vi "Car Wash.vi"() -> ()   [LabVIEW 2015]
uses:
  controls/Car Wash Indicators.ctl
  controls/Wash Options.ctl
  controls/UI Data.ctl
  support/Message Queue/Enqueue Message (Single).vi
  <vilib>/Utility/error.llb/Error Cluster From Error Code.vi
  <vilib>/ErrorRing/Error Ring.xnode
  support/Message Queue/Message Queue.lvlib
  support/User Event - Stop/User Event - Stop.lvlib
panel:
  in  "Start":bool
  out "Elapsed Time":dbl format="%0.2f"
  in  "stop":bool
  out "Wash Entry":bool
  in  "Wash Options":T1
  in  "Car Position Slider":u8(slide) max=3 scale=0.0..4.0
  out "Car Wash Indicators":T2
  # "Entry Console"
  # "Car Wash Display"
  # "Car Position Simulation"
  # "Pre-Soak\nH-P Wash\nL-P Wax\nSpot Free Rinse"
  # "Underbody Wash\nBug Remover"
  # "Tire Shine\nAir Dry"
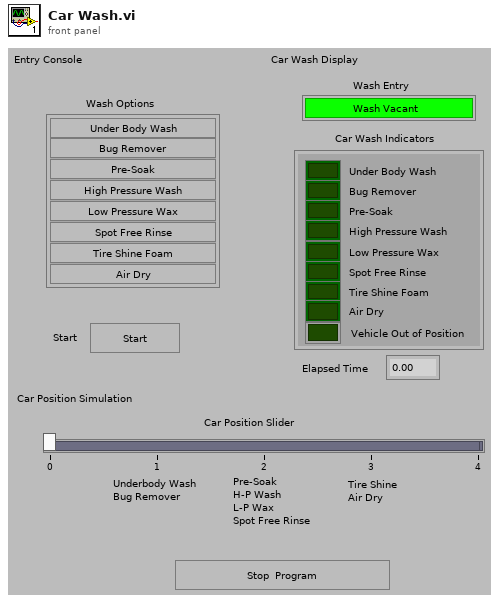
[diagram p1: front panel]
types:
  T1 = typedef "Wash Options.ctl" = cluster{"Underbody Wash":bool, "Bug Remover":bool, "Pre-Soak":bool, "High Pressure Wash":bool, "Low Pressure Wax":bool, "Spot Free Rinse":bool, "Tire Shine Foam":bool, "Air Dry":bool}
  T2 = typedef "Car Wash Indicators.ctl" = cluster{"Under Body Wash":bool, "Bug Remover":bool, "Pre-Soak":bool, "High Pressure Wash":bool, "Low Pressure Wax":bool, "Spot Free Rinse":bool, "Tire Shine Foam":bool, "Air Dry":bool, "Vehicle Out of Position":bool}
  T3 = typedef "UI Data.ctl" = cluster{"Underbody Wash Ref":refnum<vi>, "Bug Remover Ref":refnum<vi>, "Pre-Soak Ref":refnum<vi>, "High Pressure Wash Ref":refnum<vi>, "Low Pressure Wax Ref":refnum<vi>, "Spot Free Rinse Ref":refnum<vi>, "Tire Shine Foam Ref":refnum<vi>, "Air Dry Ref":refnum<vi>}
  T4 = typedef "Message Queue.lvlib/All Message Queues.ctl" = cluster{"UI":refnum<queue>}
  T5 = enum8{"Enabled", "Disabled", "Disabled and Grayed Out"}
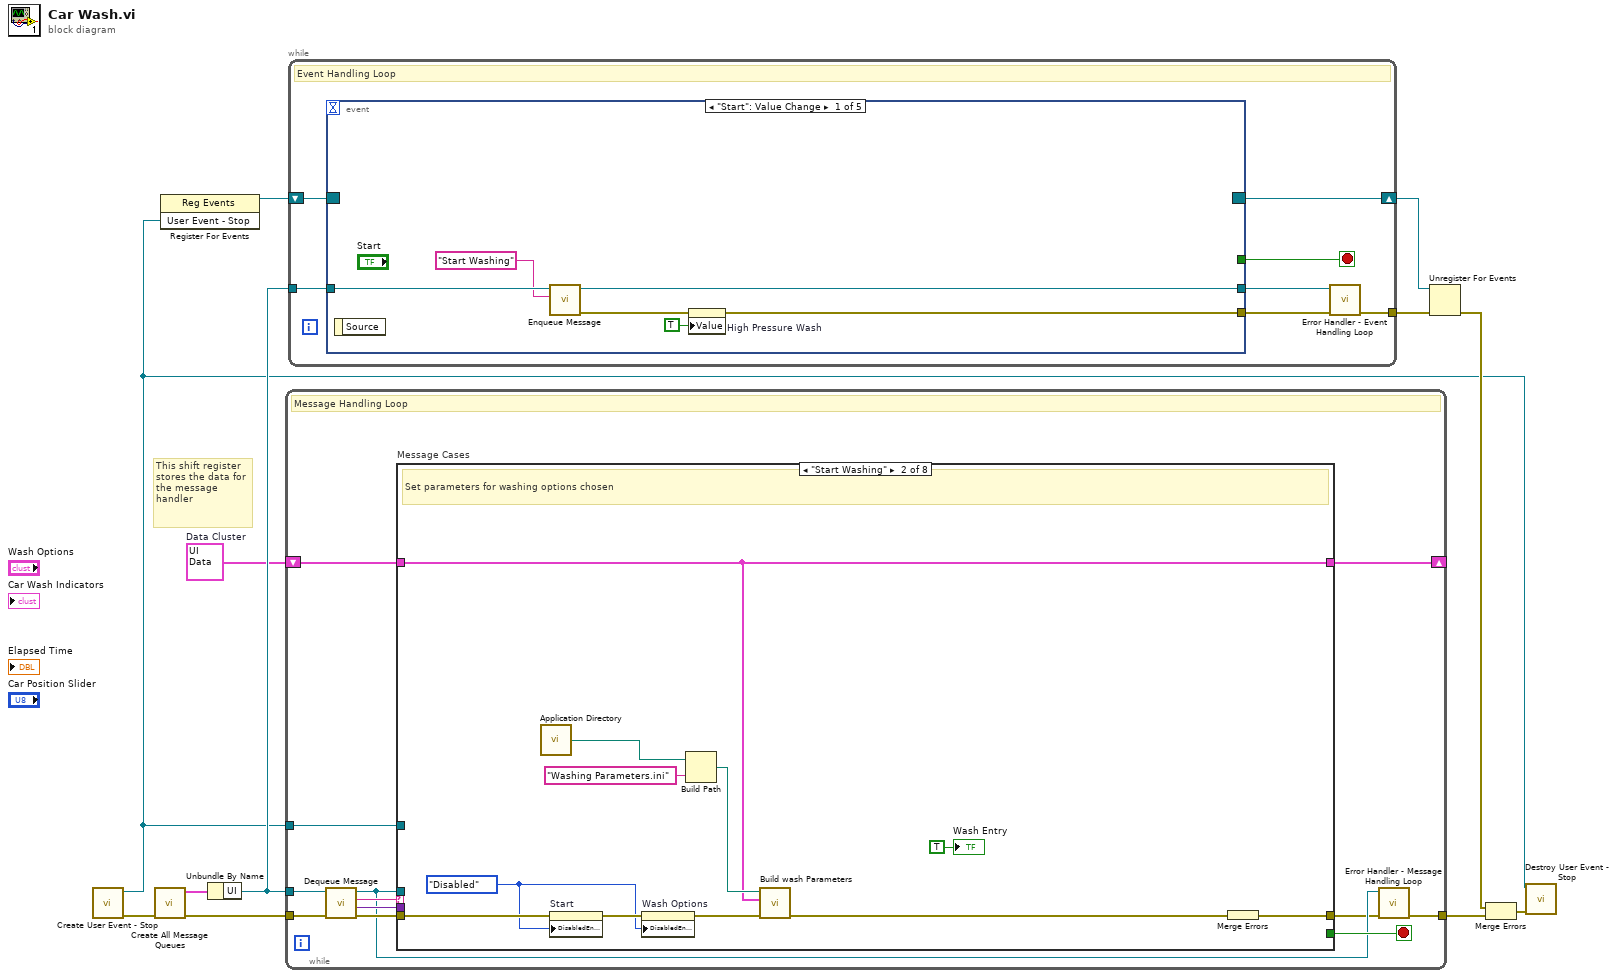
[diagram p0: block diagram]
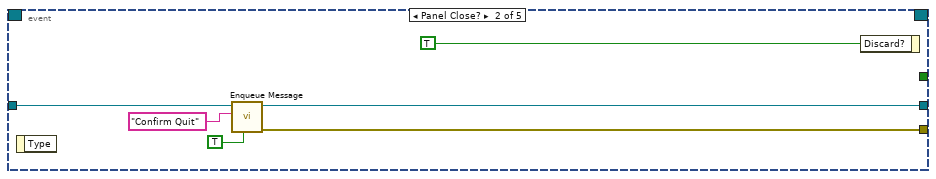
[diagram p2: hidden frame]
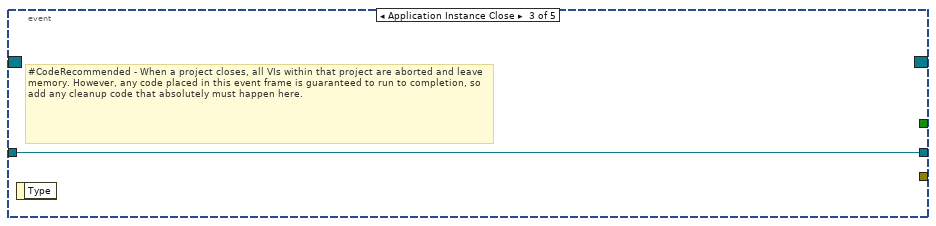
[diagram p3: hidden frame]
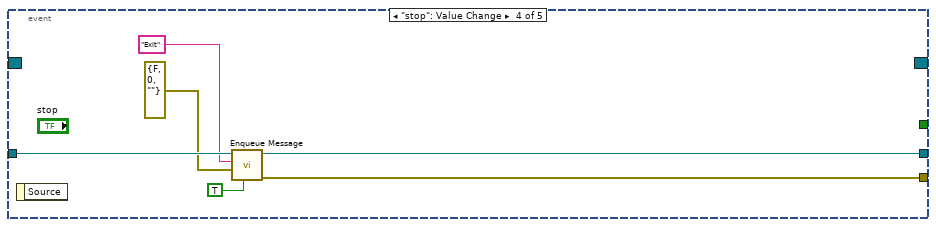
[diagram p4: hidden frame]
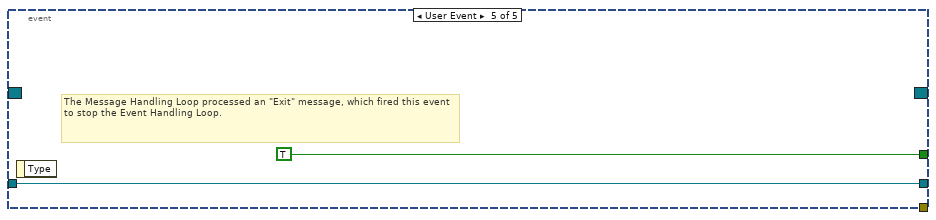
[diagram p5: hidden frame]
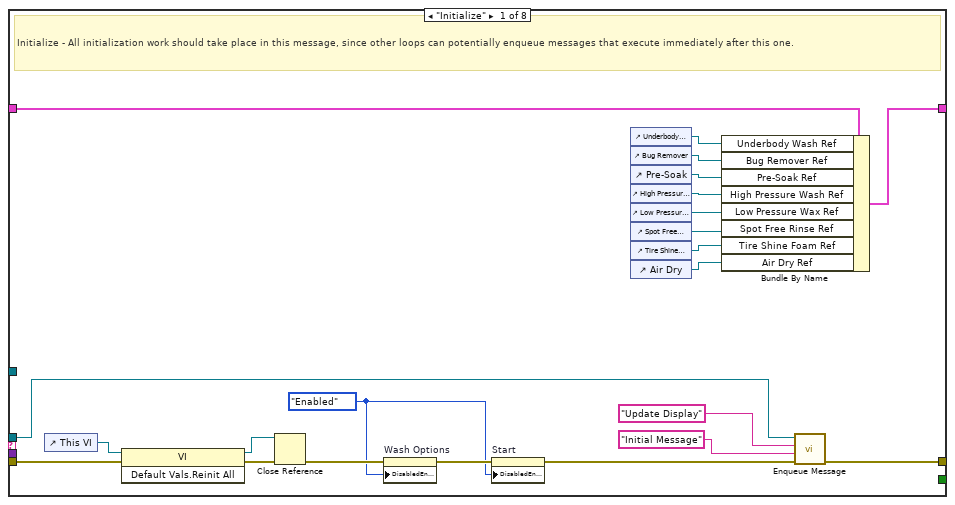
[diagram p6: hidden frame]
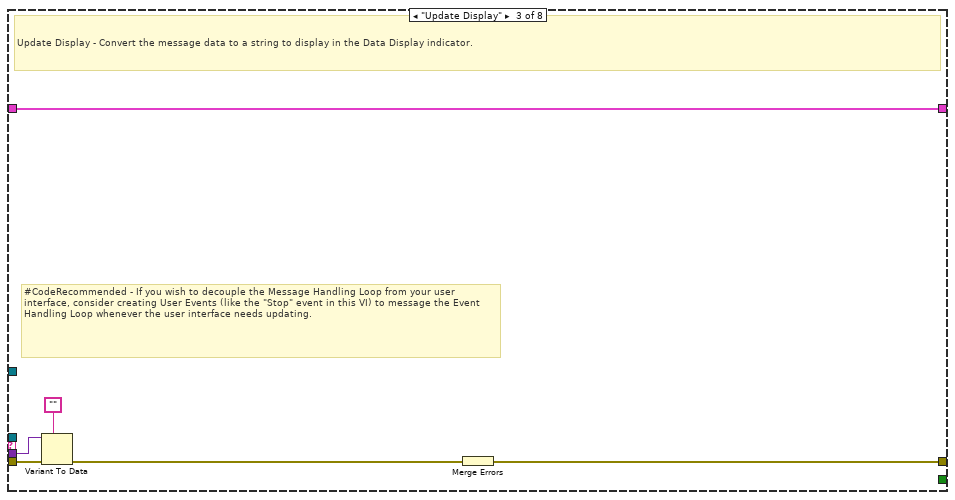
[diagram p7: hidden frame]
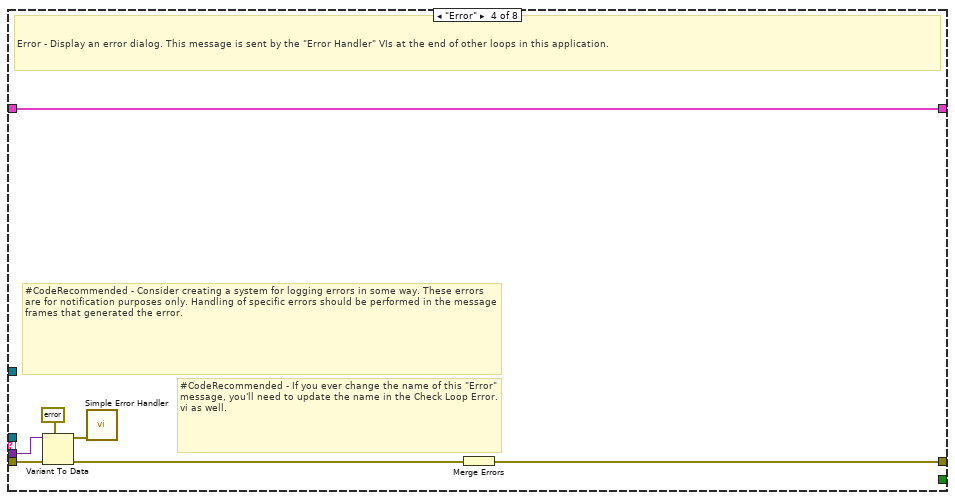
[diagram p8: hidden frame]
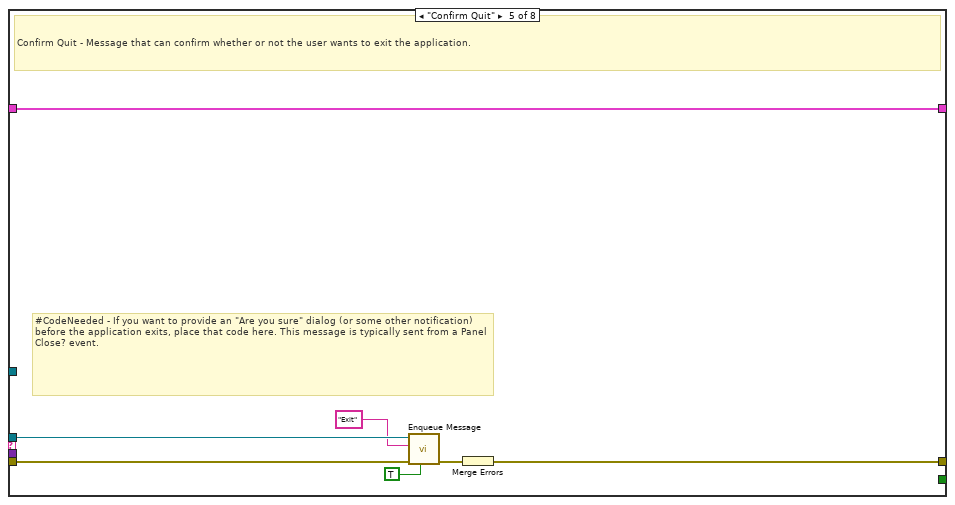
[diagram p9: hidden frame]
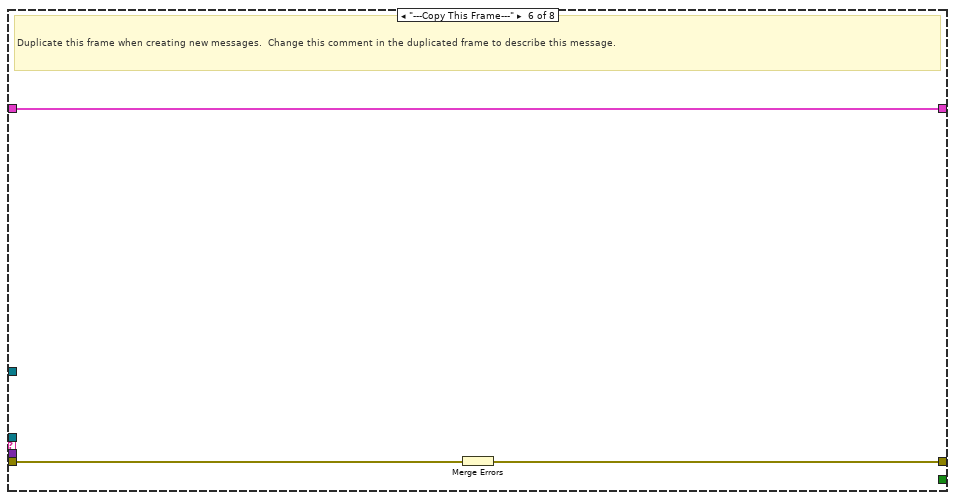
[diagram p10: hidden frame]
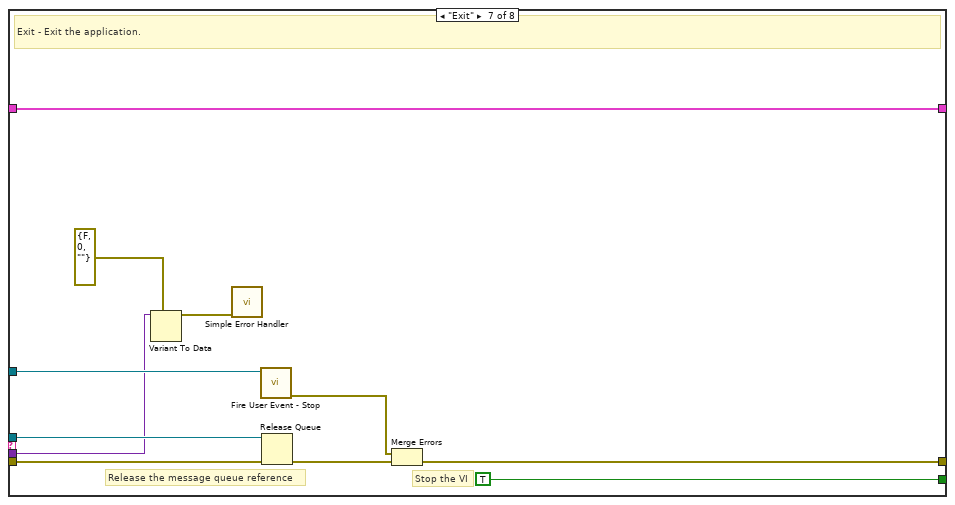
[diagram p11: hidden frame]
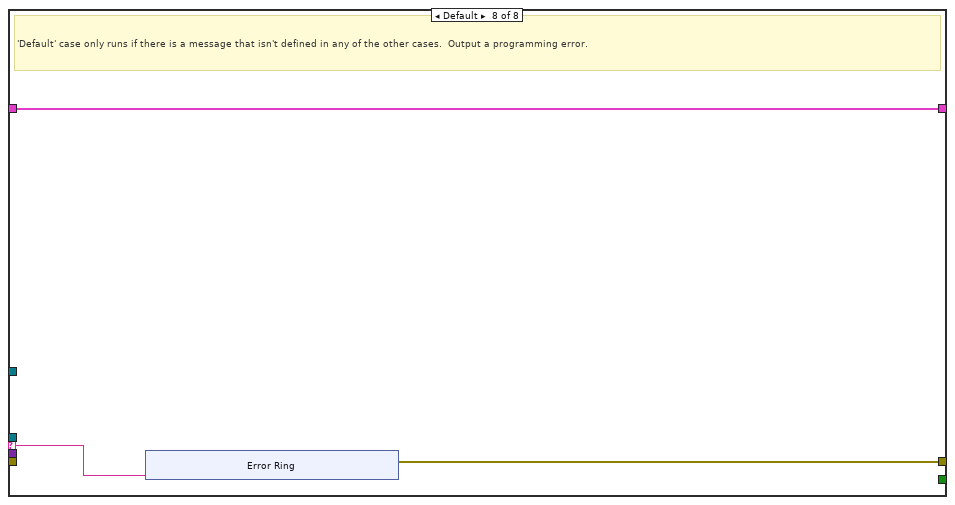
[diagram p12: hidden frame]
diagram:
  w4 = T3 {"Underbody Wash Ref"=refnum, "Bug Remover Ref"=refnum, "Pre-Soak Ref"=refnum, "High Pressure Wash Ref"=refnum, "Low Pressure Wax Ref"=refnum, "Spot Free Rinse Ref"=refnum, "Tire Shine Foam Ref"=refnum, "Air Dry Ref"=refnum}  # Data Cluster
  # "This shift register stores the data for the message handler"
  n1 = call "Create User Event - Stop.vi"() -> ("error out"=w8:errorcluster, "User Event - Stop"=w1:refnum<user-event>)  [unwired: 10 in]
  n2 = call "Create All Message Queues.vi"("error in (no error)"=w8) -> ("error out"=w12:errorcluster, "Message Queues out"=w11:T4)  [unwired: 9 in]
  n3 = register-events(w1) -> (reference out=w2:refnum<event-registration>)  [unwired: 2 in, 1 out]
  n4 = Unbundle By Name(w11) -> ("UI"=w9:refnum<queue>)
  n5 = while {
    tunnel: w9 -> [w16]
    shift-right: [w23] -> _
    shift-left: w4 -> [w24]
    tunnel: w1 -> [w21]
    tunnel: w12 -> [w20]
    tunnel: [w14] -> w10
    stop <- w22 stop-if-true
    # "Message Handling Loop"
    n6 = call "Dequeue Message.vi"("error in (no error)"=w20, "Message Queue"=w16) -> ("error out"=w19:errorcluster, "Message Data"=w17:variant, "Message"=w18:string, "dup Message Queue"=w15:refnum<queue>)  [unwired: 6 in]
    n7 = case "Message Cases" shown="\"Start Washing\"" w18 {
      selector: w18 -> [_ _ _ _ _ _ _ w92]
      tunnel: w15 -> [w44 _ _ _ w73 _ w91 _]
      tunnel: w19 -> [w31 w49 w61 w70 w77 w80 w84 _]
      tunnel: [w46 w57 w62 w64 w75 w78 w87 w93] -> w13
      tunnel: w24 -> [w34 w53 w63 w69 w76 w79 w90 w94]
      tunnel: [w33 w53 w63 w69 w76 w79 w90 w94] -> w23
      tunnel: [_ _ _ _ _ _ TRUE _] -> w22
      tunnel: w17 -> [_ _ w60 w68 _ _ w82 _]
      tunnel: w21 -> [_ _ _ _ _ _ w86 _]
      frame "Initialize" {
        w26 = T5."Enabled" ("Disabled")
        # "Initialize - All initialization work should take place in this message, since other loops can potentially enqueue messages that execute immediately after this one."
        n8 = control-ref of="This VI"() -> (w32:refnum<vi>)
        n9 = invoke class="VI" method="Default Vals.Reinit All"(reference=w32, error in=w31) -> (reference out=w30:refnum<vi>, error out=w29:errorcluster)  [unwired: 1 in, 1 out]
        n10 = Close Reference(reference=w30, error in (no error)=w29) -> (error out=w28:errorcluster)
        n11 = property on="Wash Options" class="Clust (strict)"(error in=w28, "DisabledEnum"=w26) -> (error out=w27:errorcluster)  [unwired: 1 in, 1 out]
        n12 = property on="Start" class="Bool"(error in=w27, "DisabledEnum"=w26) -> (error out=w25:errorcluster)  [unwired: 1 in, 1 out]
        n13 = control-ref of="Underbody Wash"() -> (w42:refnum<vi>)
        n14 = control-ref of="Bug Remover"() -> (w41:refnum<vi>)
        n15 = control-ref of="Pre-Soak"() -> (w40:refnum<vi>)
        n16 = control-ref of="High Pressure Wash"() -> (w39:refnum<vi>)
        n17 = control-ref of="Low Pressure Wax"() -> (w38:refnum<vi>)
        n18 = control-ref of="Spot Free Rinse"() -> (w37:refnum<vi>)
        n19 = control-ref of="Tire Shine Foam"() -> (w36:refnum<vi>)
        n20 = control-ref of="Air Dry"() -> (w35:refnum<vi>)
        n21 = Bundle By Name(cluster=w34, "Underbody Wash Ref"=w42, "Bug Remover Ref"=w41, "Pre-Soak Ref"=w40, "High Pressure Wash Ref"=w39, "Low Pressure Wax Ref"=w38, "Spot Free Rinse Ref"=w37, "Tire Shine Foam Ref"=w36, "Air Dry Ref"=w35) -> (w33:T3)
        n22 = call-poly "Enqueue Message.vi"("error in (no error)"=w25, "Message Data"="Initial Message" ("Initial Message"), "Message"="Update Display", "Message Queue"=w44) -> ("error out"=w46:errorcluster)  [unwired: 6 in, 1 out]
      }
      frame "Start Washing" {
        w48 = T5."Disabled" ("Disabled")
        # "Set parameters for washing options chosen"
        n23 = call <vilib>:"Application Directory.vi"() -> ("Application Directory"=w56:path)
        n24 = property on="Start" class="Bool"(error in=w49, "DisabledEnum"=w48) -> (error out=w50:errorcluster)  [unwired: 1 in, 1 out]
        n25 = property on="Wash Options" class="Clust (strict)"(error in=w50, "DisabledEnum"=w48) -> (error out=w51:errorcluster)  [unwired: 1 in, 1 out]
        n26 = Build Path(base path=w56, name or relative path="Washing Parameters.ini") -> (appended path=w54:path)
        n27 = call "Build wash Parameters.vi"("error in (no error)"=w51, "Data Controls"=w53, "configuration file path"=w54) -> ("error out"=w52:errorcluster)  [unwired: 7 in, 1 out]
        n28 = Merge Errors(w52) -> (w57:errorcluster)
        "Wash Entry" <- TRUE ("Wash Entry")
      }
      frame "Update Display" {
        # "#CodeRecommended - If you wish to decouple the Message Handling Loop from your user interface, consider creating User Events (like the \"Stop\" event in this VI) to message the Event Handling Loop whenever the user interface needs updating."
        # "Update Display - Convert the message data to a string to display in the Data Display indicator."
        n29 = Variant To Data(error in=w61, type="", Variant=w60) -> (error out=w58:errorcluster)  [unwired: 1 out]
        n30 = Merge Errors(w58) -> (w62:errorcluster)
      }
      frame "Error" {
        # "#CodeRecommended - If you ever change the name of this \"Error\" message, you'll need to update the name in the Check Loop Error.vi as well."
        # "#CodeRecommended - Consider creating a system for logging errors in some way. These errors are for notification purposes only. Handling of specific errors should be performed in the message frames that generated the error."
        # "Error - Display an error dialog. This message is sent by the \"Error Handler\" VIs at the end of other loops in this application."
        n31 = Variant To Data(error in=w70, type=errorcluster {"status"=FALSE, "code"=0, "source"=""} ("error constant"), Variant=w68) -> (data=w66:errorcluster, error out=w65:errorcluster)
        n32 = call <vilib>:"Simple Error Handler.vi"("error in (no error)"=w66) -> ()  [unwired: 4 in, 5 out]
        n33 = Merge Errors(w65) -> (w64:errorcluster)
      }
      frame "Confirm Quit" {
        # "#CodeNeeded - If you want to provide an \"Are you sure\" dialog (or some other notification) before the application exits, place that code here. This message is typically sent from a Panel Close? event."
        # "Confirm Quit - Message that can confirm whether or not the user wants to exit the application."
        n34 = call-poly "Enqueue Message.vi"("Priority Message? (F)"=TRUE, "error in (no error)"=w77, "Message"="Exit", "Message Queue"=w73) -> ("error out"=w74:errorcluster)  [unwired: 6 in, 1 out]
        n35 = Merge Errors(w74) -> (w75:errorcluster)
      }
      frame "---Copy This Frame---" {
        # "Duplicate this frame when creating new messages.  Change this comment in the duplicated frame to describe this message."
        n36 = Merge Errors(w80) -> (w78:errorcluster)
      }
      frame "Exit" {
        # "Stop the VI"
        # "Release the message queue reference"
        # "Exit - Exit the application."
        n37 = Variant To Data(type=errorcluster {"status"=FALSE, "code"=0, "source"=""} ("error out"), Variant=w82) -> (data=w81:errorcluster)  [unwired: 1 in, 1 out]
        n38 = call <vilib>:"Simple Error Handler.vi"("error in (no error)"=w81) -> ()  [unwired: 4 in, 5 out]
        n39 = call "Fire User Event - Stop.vi"("User Event - Stop"=w86) -> ("error out"=w85:errorcluster)  [unwired: 10 in]
        n40 = Release Queue(queue=w91, error in (no error)=w84) -> (error out=w88:errorcluster)  [unwired: 1 in, 2 out]
        n41 = Merge Errors(w85, w88) -> (w87:errorcluster)
      }
      frame Default {
        # "'Default' case only runs if there is a message that isn't defined in any of the other cases.  Output a programming error."
        n42 = xnode "Error Ring"("parameter 0"=w92) -> ("error out"=w93:errorcluster)
      }
    }
    n43 = call "Error Handler - Message Handling Loop.vi"("error in (no error)"=w13, "Message Queue"=w15) -> ("dup error in"=w14:errorcluster)  [unwired: 8 in, 1 out]
  }
  n44 = while {
    tunnel: w9 -> [w108]
    shift-right: [w106] -> w5
    shift-left: w2 -> [w107]
    tunnel: [w102] -> w3
    stop <- w104 stop-if-true
    # "Event Handling Loop"
    n45 = event shown="[0] \"Start\": Value Change" {
      selector: w107 -> [_ _ _ _ _]
      dyn-events: [_ _ _ _ _] -> w106
      timeout: _ -> [_ _ _ _ _]
      tunnel: [_ _ _ _ TRUE ("Discard?")] -> w104
      tunnel: w108 -> [w114 w119 w121 w127 w129]
      tunnel: [w110 w118 _ w126 _] -> w105
      tunnel: [w113 w117 w121 w125 w129] -> w103
      event "Start": Value Change {
        n46 = event-data() -> ()  [unwired: 1 in, 1 out]
        n47 = call-poly "Enqueue Message.vi"("Message"="Start Washing", "Message Queue"=w114) -> ("error out"=w111:errorcluster, "dup Message Queue"=w113:refnum<queue>)  [unwired: 8 in]
        n48 = property on="High Pressure Wash" class="Bool (strict)"(error in=w111, "Value"=TRUE) -> (error out=w110:errorcluster)  [unwired: 1 in, 1 out]
      }
      event Panel Close? {
        n49 = event-data() -> ()  [unwired: 1 in, 1 out]
        n50 = call-poly "Enqueue Message.vi"("Priority Message? (F)"=TRUE, "Message"="Confirm Quit", "Message Queue"=w119) -> ("error out"=w118:errorcluster, "dup Message Queue"=w117:refnum<queue>)  [unwired: 7 in]
        n51 = event-data("Discard?"=TRUE) -> ()  [unwired: 1 in, 1 out]
      }
      event Application Instance Close {
        # "#CodeRecommended - When a project closes, all VIs within that project are aborted and leave memory. However, any code placed in this event frame is guaranteed to run to completion, so add any cleanup code that absolutely must happen here."
        n52 = event-data() -> ()  [unwired: 1 in, 1 out]
      }
      event "stop": Value Change {
        n53 = event-data() -> ()  [unwired: 1 in, 1 out]
        n54 = call-poly "Enqueue Message.vi"("Priority Message? (F)"=TRUE, "Message Data"=errorcluster {"status"=FALSE, "code"=0, "source"=""} ("error out"), "Message"="Exit", "Message Queue"=w127) -> ("error out"=w126:errorcluster, "dup Message Queue"=w125:refnum<queue>)  [unwired: 6 in]
      }
      event User Event {
        # "The Message Handling Loop processed an \"Exit\" message, which fired this event to stop the Event Handling Loop."
        n55 = event-data() -> ()  [unwired: 1 in, 1 out]
      }
    }
    n56 = call "Error Handler - Event Handling Loop.vi"("error in (no error)"=w105, "Message Queue"=w103) -> ("dup error in"=w102:errorcluster)  [unwired: 8 in, 1 out]
  }
  n57 = Unregister For Events(event registration refnum=w5, error in=w3) -> (error out=w6:errorcluster)
  n58 = Merge Errors(w6, w10) -> (w7:errorcluster)
  n59 = call "Destroy User Event - Stop.vi"("error in (no error)"=w7, "User Event - Stop"=w1) -> ()  [unwired: 9 in, 1 out]
